vi "Set_IP_Simulation_Status.vi"(8 "error in (no error)":errorcluster, 9 "Cellular Tech":string="ip_simulation", 10 "value":i32 min=0 max=1, 11 "Base Station":T1) -> (0 "error out":errorcluster, 3 "Output String":string)   [LabVIEW 2021]
uses:
  Controls/Base_Station_Emulator.ctl
  Controls/TCP_FGV.ctl
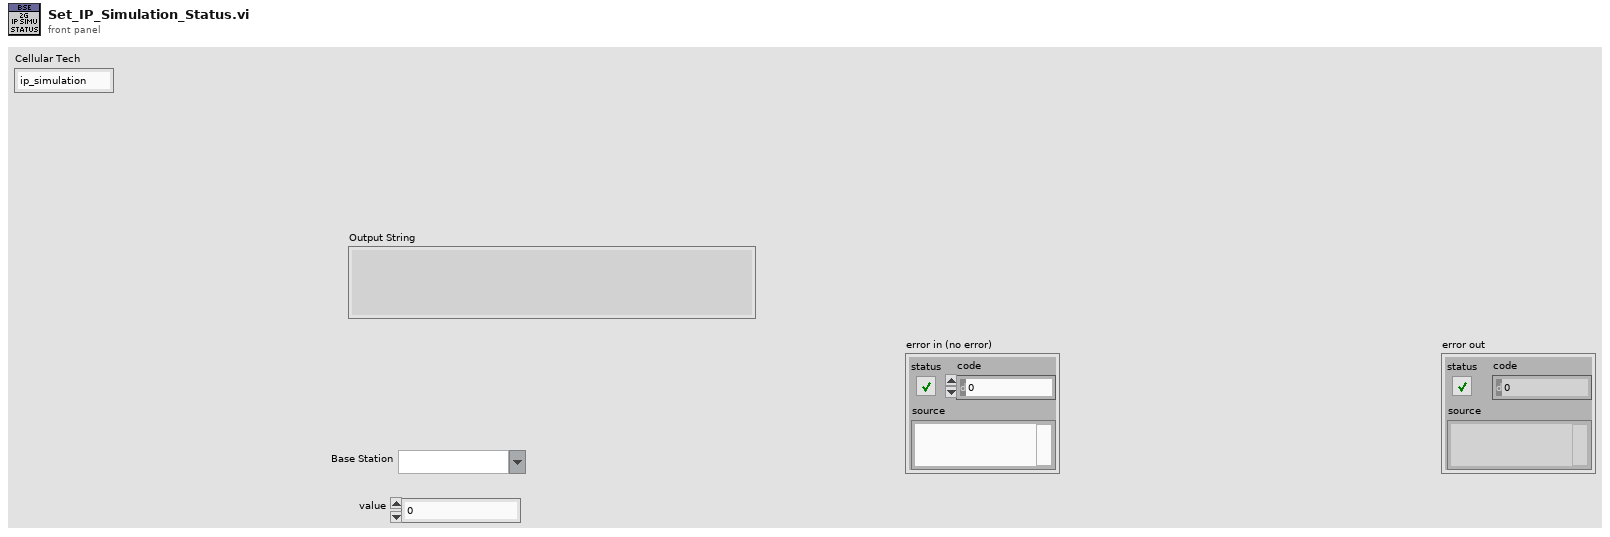
[diagram p1: front panel]
types:
  T1 = typedef "Base_Station_Emulator.ctl" = string
  T2 = typedef "TCP_FGV.ctl" = enum16{"Open", "Read", "Write", "Close"}
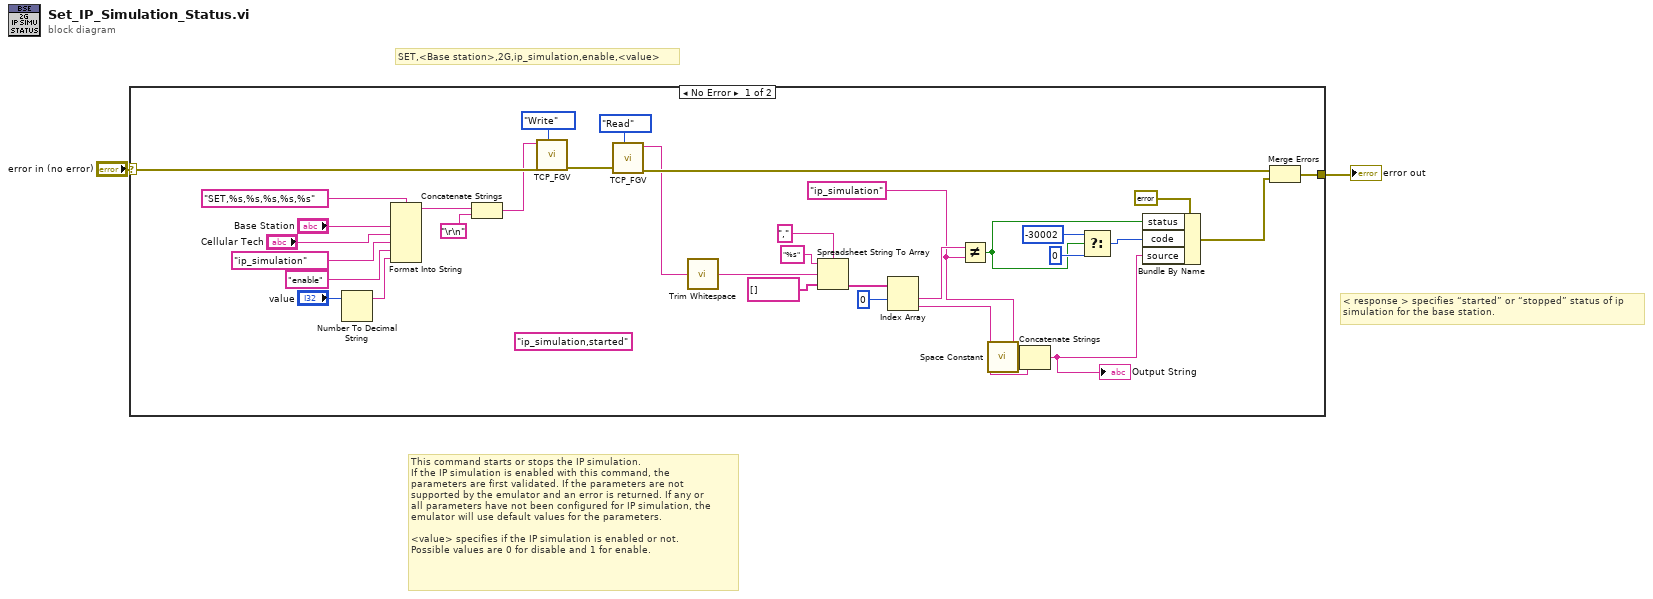
[diagram p0: block diagram]
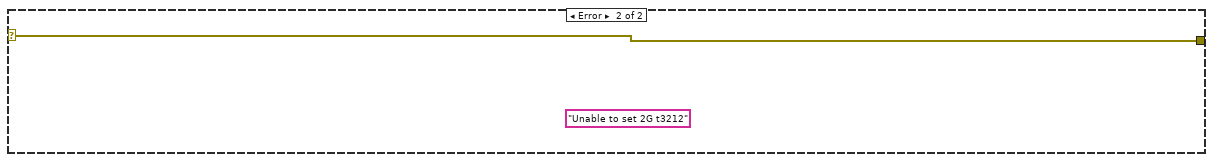
[diagram p2: hidden frame]
diagram:
  # "< response > specifies “started” or “stopped” status of ip \nsimulation for the base station."
  # "This command starts or stops the IP simulation. \nIf the IP simulation is enabled with this command, the \nparameters are first validated. If the parameters are not \nsupported by the emulator and an error is returned. If any or \nall parameters have not been configured for IP simulation, the\nemulator will use default values for the parameters.  \n\n<value> specifies if the IP simulation is enabled or not. \nPossible values are 0 for disable and 1 for enable."
  # "SET,<Base station>,2G,ip_simulation,enable,<value>"
  n1 = case shown="No Error" "error in (no error)" {
    selector: "error in (no error)" -> [w33 w37]
    tunnel: [w18 w37] -> w1
    frame No Error {
      (unwired) "ip_simulation,started" ("format string")
      w7 = "ip_simulation" ("format string")
      n2 = Number To Decimal String(number="value") -> (decimal integer string=w12:string)  [unwired: 1 in]
      n3 = Format Into String(format string="SET,%s,%s,%s,%s,%s", "Base Station", "Cellular Tech", "ip_simulation", "enable", w12) -> (resulting string=w10:string)  [unwired: 2 in, 1 out]
      n4 = Concatenate Strings(w10, "\r\n") -> (w9:string)
      n5 = call "TCP_FGV.vi"("Command"=w9, "error in (no error)"=w33, "Operation"=TCP_FGV."Write") -> ("error out"=w19:errorcluster)  [unwired: 6 in, 1 out]
      n6 = call "TCP_FGV.vi"("error in (no error)"=w19, "Operation"=TCP_FGV."Read") -> ("Data Out"=w4:string, "error out"=w21:errorcluster)  [unwired: 7 in]
      n7 = call <vilib>:"Trim Whitespace.vi"("string"=w4) -> ("trimmed string"=w30:string)  [unwired: 1 in]
      n8 = Spreadsheet String To Array(delimiter (Tab)=",", format string="%s", spreadsheet string=w30, array type (2D Dbl)=string[] []) -> (array=w29:string[])
      n9 = Index Array(array=w29, index #1=0 ("index")) -> (element #1=w22:string, element #2=w16:string)  [unwired: 1 in]
      n10 = Not Equal?(x=w22, y=w7) -> (x != y?=w5:bool)
      n11 = call <vilib>:"Space Constant.vi"() -> ("String"=w17:string)
      n12 = Concatenate Strings(w7, w17, w16) -> (w15:string)
      "Output String" <- w15
      n13 = Select(t=-30002 ("code"), s=w5, f=0 ("code")) -> (s? t:f=w31:i32)
      n14 = Bundle By Name(cluster=errorcluster {"status"=FALSE, "code"=0, "source"=""} ("error constant"), "status"=w5, "code"=w31, "source"=w15) -> (w20:errorcluster)
      n15 = Merge Errors(w21, w20) -> (w18:errorcluster)
    }
    frame Error {
      (unwired) "Unable to set 2G t3212" ("source")
    }
  }
  "error out" <- w1
